vi "objToPointer.vi"(10 "objIn":refnum<class>) -> (2 "stringOut":string)   [LabVIEW 2009]
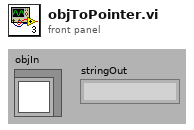
[diagram p1: front panel]
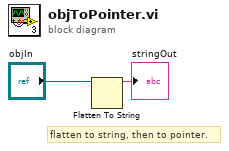
[diagram p0: block diagram]
diagram:
  # "flatten to string, then to pointer."
  n1 = Flatten To String(anything="objIn") -> (data string=→"stringOut":string)  [unwired: 3 in, 2 out]
